vi "Flush and Clear.vi"(8 "error in (no error)":errorcluster, 11 "Sequencer in":refnum<class "Sequencer.lvclass">) -> (0 "error out":errorcluster, 3 "Sequencer out":refnum<class "Sequencer.lvclass">)   [LabVIEW 2020, in "Sequencer.lvlib" / "Sequencer.lvclass"]
doc: "Flush the Sequencer Core and cancel any notification on the interrupt notifier."
uses:
  Sequencer.lvclass
  Sequencer.lvclass/Sequencer.ctl
  Sequencer Core/Sequencer Core.lvclass/Sequencer Core.ctl
  PPL/HDH.Data.Generic.lvlibp/Synchronization/Notifier/Cancel.vi
  Message Priority Queue/Flush.vi
  Sequencer Core/Sequencer Core.lvclass
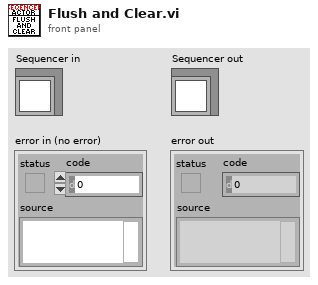
[diagram p1: front panel]
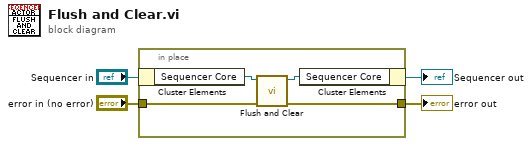
[diagram p0: block diagram]
diagram:
  n1 = in-place {
    in-place-border: "error in (no error)" -> [w6]
    in-place-border: [w5] -> w1
    n2 = in-place-cluster #1("Sequencer in") -> ("Sequencer Core"=w8:refnum<class "Sequencer Core.lvclass">)
    n3 = call "Flush and Clear.vi"("error in (no error)"=w6, "Sequencer Core in"=w8) -> ("error dub"=w5:errorcluster, "Sequencer Core out"=w7:refnum<class "Sequencer Core.lvclass">)  [unwired: 8 in]
    n4 = in-place-cluster #1("Sequencer Core"=w7) -> (→"Sequencer out":refnum<class "Sequencer.lvclass">)
  }
  "error out" <- w1
